vi "PowerLawFit.vi"(5 "MinFitZ":dbl, 7 "MaxFitZ":dbl, 8 "ZeroDisplacement?":enum16{"Allow d0", "No displacement"}(ring), 9 "Zref":dbl, 10 "U/Uref":dbl[](array[numeric]), 11 "z":dbl[](array[numeric])) -> (0 "PowerLaw":cluster{"n":dbl, "d0":dbl}, 1 "PowerLawFitEquation":string, 2 "CroppedData":cluster{"X Out":dbl[], "Y Out":dbl[]}, 3 "FitCurve":T2)   [LabVIEW 2013]
uses:
  <vilib>/Analysis/6fits.llb/Curve Fitting Criteria.ctl
  <vilib>/Analysis/6fits.llb/Remove Outliers (Range).vi
  <vilib>/gmath/NumericalOptimization/Nonlinear Curve Fit LM formula string.vi
  <vilib>/gmath/NI_Gmath.lvlib
  <vilib>/Analysis/NI_AALPro.lvlib
panel:
  in  "noDisplacementmethod":T1=1 items=["Least Square", "Least Absolute Residual", "Bisquare"]
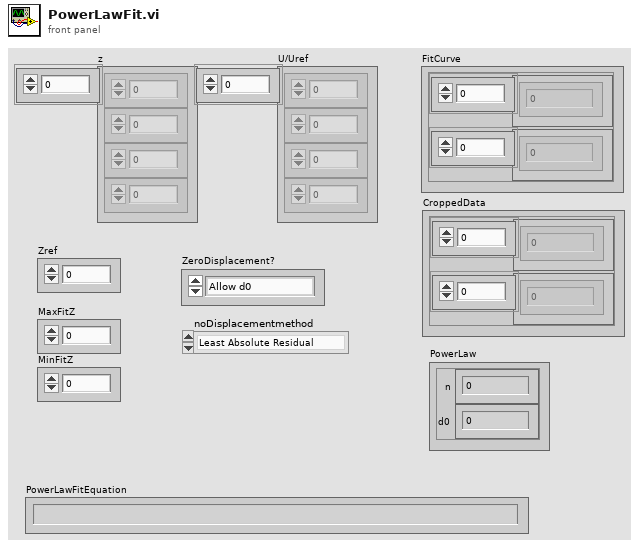
[diagram p1: front panel]
types:
  T1 = typedef "NI_AALPro.lvlib/Curve Fitting Criteria.ctl" = u16
  T2 = cluster{"Array":dbl[], "best nonlinear fit":dbl[]}
  T3 = cluster{"model":string, "Parameters":string[], "x":string}
  T4 = cluster{"amp min":dbl, "amp max":dbl, "power min":dbl, "power max":dbl, "offset min":dbl, "offset max":dbl}
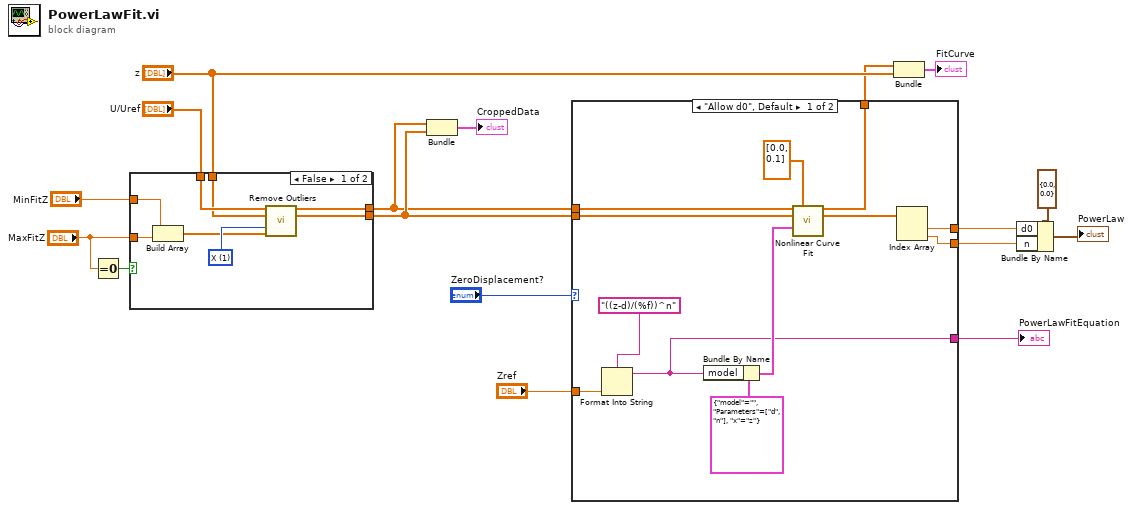
[diagram p0: block diagram]
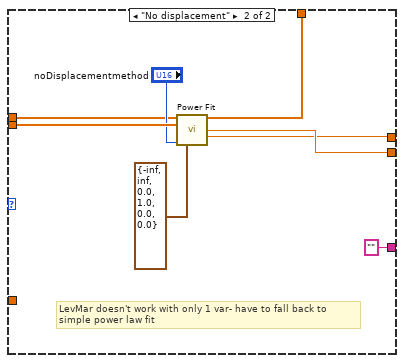
[diagram p2: hidden frame]
diagram:
  n1 = Equal To 0?(x="MaxFitZ") -> (x = 0?=w13:bool)
  n2 = case shown="False" w13 {
    tunnel: [w25 w26] -> w10
    tunnel: [w24 w27] -> w11
    tunnel: "U/Uref" -> [w22 w26]
    tunnel: "z" -> [w21 w27]
    tunnel: "MaxFitZ" -> [w19 _]
    tunnel: "MinFitZ" -> [w18 _]
    frame False {
      w23 = u16 1 items=["x", "X", "X and Y"] ("range type")
      n3 = Build Array(w18, w19) -> (w20:dbl[])
      n4 = call-poly <vilib>:"Remove Outliers.vi"("Y"=w22, "X"=w21, "range type"=w23, "Range"=w20) -> ("Y Out"=w25:dbl[], "X Out"=w24:dbl[])  [unwired: 7 in, 3 out]
    }
    frame True {
    }
  }
  n5 = Bundle("U/Uref"=w10, "z"=w11) -> (→"CroppedData":cluster{"U/Uref":dbl[], "z":dbl[]})  [unwired: 1 in]
  n6 = case shown="\"Allow d0\", Default" "ZeroDisplacement?" {
    tunnel: [w37 ""] -> w12
    tunnel: w11 -> [w36 w42]
    tunnel: w10 -> [w35 w40]
    tunnel: [w34 w44] -> w5
    tunnel: [w33 w46] -> w4
    tunnel: "Zref" -> [w32 _]
    tunnel: [w31 w47] -> w8
    frame "Allow d0", Default {
      n7 = Format Into String(format string="((z-d)/(%f))^n" ("vonKarman Spectrum"), w32) -> (resulting string=w37:string)  [unwired: 2 in, 1 out]
      n8 = Bundle By Name(cluster=T3 {"model"="", "Parameters"=["d", "n"], "x"="z"} ("model description"), "model"=w37) -> (w39:T3)
      n9 = call-poly <vilib>:"Nonlinear Curve Fit.vi"("Y"=w35, "initial parameters"=dbl[] [0.0, 0.1], "X"=w36, "model description"=w39) -> ("best nonlinear fit"=w31:dbl[], "best fit parameters"=w38:dbl[])  [unwired: 7 in, 3 out]
      n10 = Index Array(array=w38) -> (element #1=w34:dbl, element #2=w33:dbl)  [unwired: 2 in]
    }
    frame "No displacement" {
      # "LevMar doesn't work with only 1 var- have to fall back to\nsimple power law fit"
      n11 = call <vilib>:"Power Fit.vi"("Y"=w40, "X"=w42, "method"="noDisplacementmethod", "parameter bounds"=T4 {"amp min"=-inf, "amp max"=inf, "power min"=0.0, "power max"=1.0, "offset min"=0.0, "offset max"=0.0}) -> ("Best Power Fit"=w47:dbl[], "power"=w46:dbl, "offset"=w44:dbl)  [unwired: 6 in, 3 out]
    }
  }
  "PowerLawFitEquation" <- w12
  n12 = Bundle("Best Power Fit"=w8, "z"="z") -> (→"FitCurve":cluster{"Best Power Fit":dbl[], "z":dbl[]})  [unwired: 1 in]
  n13 = Bundle By Name(cluster=cluster{"n":dbl, "d0":dbl} {"n"=0.0, "d0"=0.0} ("PowerLaw"), "d0"=w5, "n"=w4) -> (→"PowerLaw":cluster{"n":dbl, "d0":dbl})
